vi "协议-重启模块.vi"() -> (3 "完整输出":string)   [LabVIEW 2013]
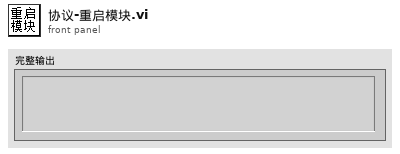
[diagram p1: front panel]
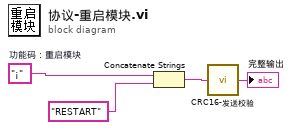
[diagram p0: block diagram]
diagram:
  w4 = "¡"  # 功能码：重启模块
  n1 = Concatenate Strings(w4, "RESTART") -> (w2:string)
  n2 = call "CRC16-发送校验.vi"("净数据"=w2) -> ("完整输出"=→"完整输出":string)
